vi "MergeAttrMap.vi"(6 "If exist? Skip(T)/Overwrite(F)":bool=TRUE, 8 "error in (no error)":errorcluster, 10 "AttrMap B":T1, 11 "AttrMap A":T1) -> (0 "error out":errorcluster, 3 "AttrMap A after B->A":T1)   [LabVIEW 2019, in "lv-apt-json-file.lvlib"]
uses:
  lv-apt-json-file.lvlib
  Typedef/Def-AttrMap.ctl
  f16f814e-f0a0-47f4-ae2a-f78fd01390a2.vi
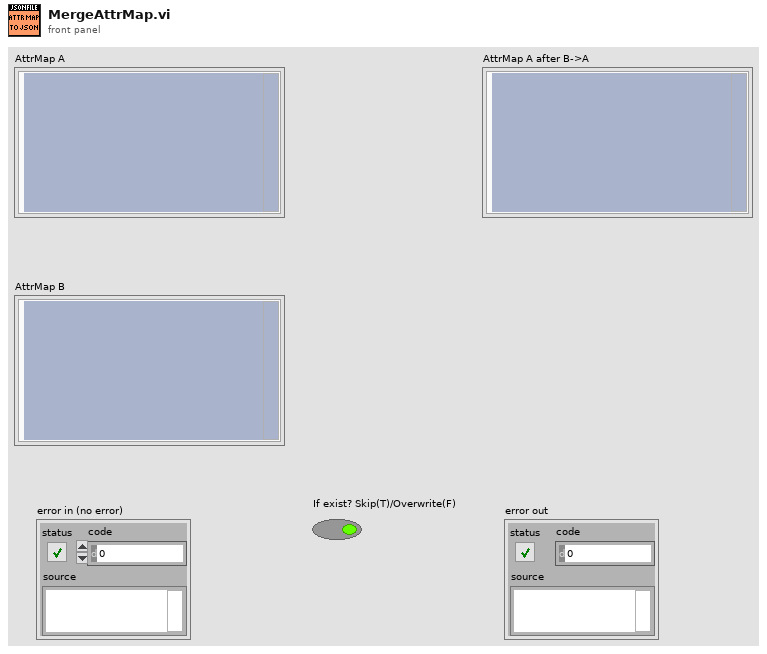
[diagram p1: front panel]
types:
  T1 = typedef "lv-apt-json-file.lvlib/Def-AttrMap.ctl" = cluster{"Map":variant}
  T2 = typedef "lv-apt-json-file.lvlib/Def-AttrMap -- Map.ctl" = map{string, string}
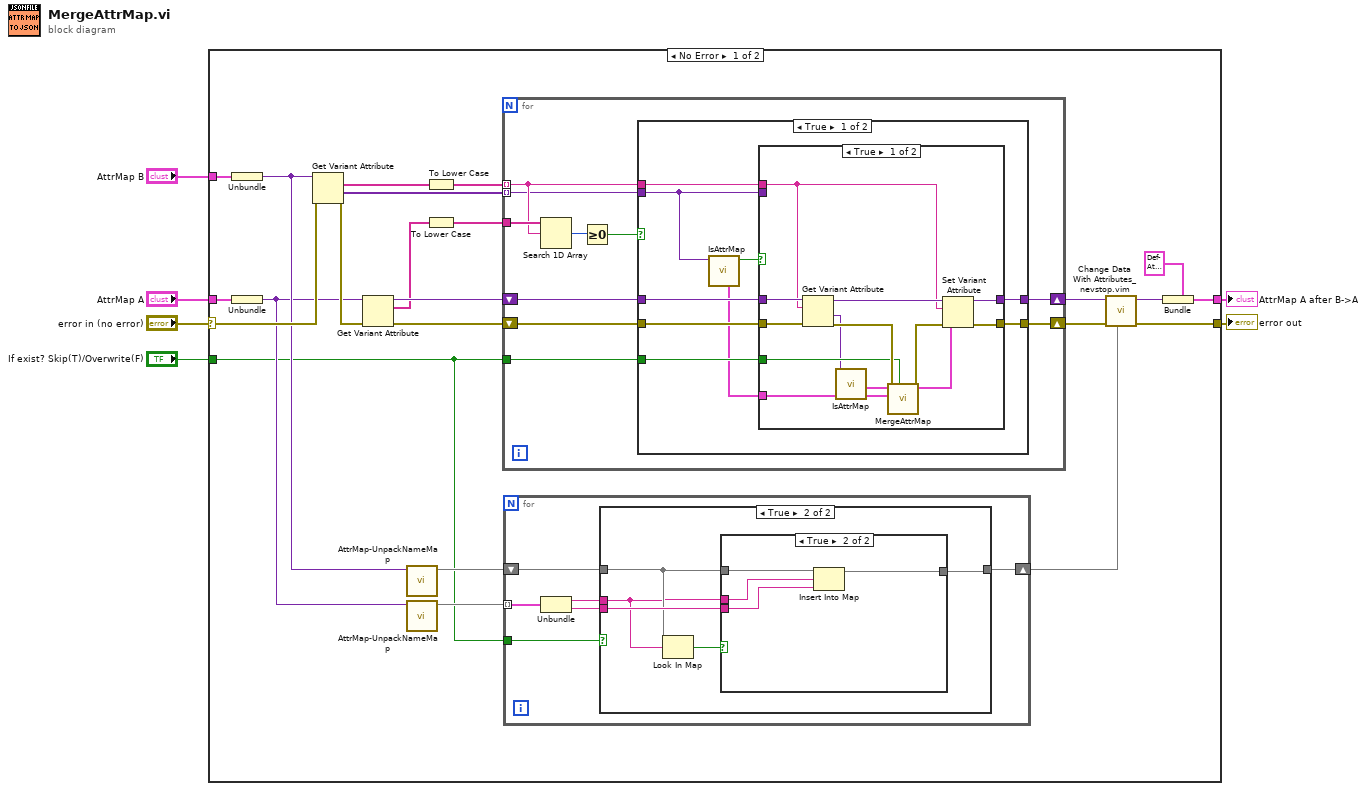
[diagram p0: block diagram]
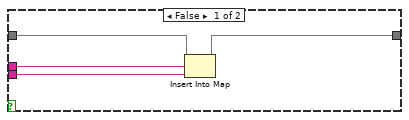
[diagram p2: hidden frame]
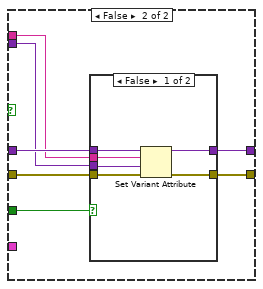
[diagram p4: hidden frame]
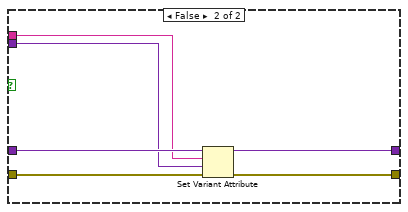
[diagram p6: hidden frame]
diagram:
  n1 = case shown="No Error" "error in (no error)" {
    selector: "error in (no error)" -> [w24 w104]
    tunnel: "AttrMap A" -> [w29 w103]
    tunnel: "AttrMap B" -> [w19 _]
    tunnel: "If exist? Skip(T)/Overwrite(F)" -> [w14 _]
    tunnel: [w9 w104] -> w2
    tunnel: [w8 w103] -> w1
    frame No Error {
      n2 = Unbundle(w19) -> ("Map"=w18:variant)
      n3 = Unbundle(w29) -> ("Map"=w17:variant)
      n4 = Get Variant Attribute(Variant=w18, error in=w24) -> (names=w21:string[], values=w22:variant[], error out=w23:errorcluster)  [unwired: 2 in, 1 out]
      n5 = Get Variant Attribute(Variant=w17, error in=w23) -> (duplicate Variant=w27:variant, names=w26:string[], error out=w28:errorcluster)  [unwired: 2 in, 1 out]
      n6 = call "AttrMap-UnpackNameMap.vi"("Map"=w18) -> ("NameMap"=w16:T2)  [unwired: 10 in]
      n7 = call "AttrMap-UnpackNameMap.vi"("Map"=w17) -> ("NameMap"=w15:T2)  [unwired: 10 in]
      n8 = To Lower Case(string=w21) -> (all lower case string=w20:string[])
      n9 = To Lower Case(string=w26) -> (all lower case string=w25:string[])
      n10 = for {
        shift-right: [w58] -> w12
        shift-left: w27 -> [w59]
        shift-right: [w56] -> w10
        shift-left: w28 -> [w57]
        tunnel: w25 -> [w55]
        tunnel: w22 -> [w51] mode=indexing
        tunnel: w20 -> [w52] mode=indexing
        tunnel: w14 -> [w50]
        n11 = Search 1D Array(1D array=w55, element=w52) -> (index of element=w54:i32)  [unwired: 1 in]
        n12 = Greater Or Equal To 0?(x=w54) -> (x >= 0?=w53:bool)
        n13 = case shown="True" w53 {
          tunnel: w59 -> [w68 w102]
          tunnel: [w67 w101] -> w58
          tunnel: w57 -> [w66 w100]
          tunnel: [w65 w99] -> w56
          tunnel: w52 -> [w62 w98]
          tunnel: w51 -> [w61 w97]
          tunnel: w50 -> [w63 _]
          frame True {
            n14 = call "IsAttrMap.vi"("Variant"=w61) -> ("True"=w64:bool, "AttrMap"=w60:T1)  [unwired: 8 in, 1 out]
            n15 = case shown="True" w64 {
              tunnel: w68 -> [w81 w88]
              tunnel: [w79 w87] -> w67
              tunnel: w66 -> [w80 w86]
              tunnel: [w78 w85] -> w65
              tunnel: w63 -> [w72 w84]
              tunnel: w62 -> [w75 w83]
              tunnel: w61 -> [_ w82]
              tunnel: w60 -> [w69 _]
              frame True {
                n16 = Get Variant Attribute(Variant=w81, name=w75, error in=w80) -> (duplicate Variant=w77:variant, value=w71:variant, error out=w74:errorcluster)  [unwired: 1 in, 1 out]
                n17 = call "IsAttrMap.vi"("Variant"=w71) -> ("AttrMap"=w70:T1)  [unwired: 8 in, 2 out]
                n18 = call "MergeAttrMap.vi"("If exist? Skip(T)/Overwrite(F)"=w72, "error in (no error)"=w74, "AttrMap B"=w69, "AttrMap A"=w70) -> ("error out"=w73:errorcluster, "AttrMap A after B->A"=w76:T1)  [unwired: 6 in]
                n19 = Set Variant Attribute(Variant=w77, name=w75, value=w76, error in=w73) -> (Variant out=w79:variant, error out=w78:errorcluster)  [unwired: 1 out]
              }
              frame False {
                n20 = case shown="False" w84 {
                  tunnel: w88 -> [w94 w96]
                  tunnel: [w93 w96] -> w87
                  tunnel: w86 -> [w92 w95]
                  tunnel: [w91 w95] -> w85
                  tunnel: w83 -> [w90 _]
                  tunnel: w82 -> [w89 _]
                  frame False {
                    n21 = Set Variant Attribute(Variant=w94, name=w90, value=w89, error in=w92) -> (Variant out=w93:variant, error out=w91:errorcluster)  [unwired: 1 out]
                  }
                  frame True {
                  }
                }
              }
            }
          }
          frame False {
            n22 = Set Variant Attribute(Variant=w102, name=w98, value=w97, error in=w100) -> (Variant out=w101:variant, error out=w99:errorcluster)  [unwired: 1 out]
          }
        }
      }
      n23 = for {
        tunnel: w15 -> [w33] mode=indexing
        shift-right: [w30] -> w13
        shift-left: w16 -> [w34]
        tunnel: w14 -> [w35]
        n24 = Unbundle(w33) -> (w32:string, w31:string)
        n25 = case shown="True" w35 {
          tunnel: w34 -> [w39 w42]
          tunnel: w32 -> [w38 w40]
          tunnel: w31 -> [w37 w43]
          tunnel: [w36 w41] -> w30
          frame False {
            n26 = Insert Into Map(map in=w39, key=w38, value=w37) -> (map out=w36:T2)  [unwired: 2 out]
          }
          frame True {
            n27 = Look In Map(map=w42, key=w40) -> (key not found?=w44:bool)  [unwired: 1 in, 1 out]
            n28 = case shown="True" w44 {
              tunnel: w43 -> [_ w47]
              tunnel: w42 -> [w45 w49]
              tunnel: [w45 w48] -> w41
              tunnel: w40 -> [_ w46]
              frame False {
              }
              frame True {
                n29 = Insert Into Map(map in=w49, key=w46, value=w47) -> (map out=w48:T2)  [unwired: 2 out]
              }
            }
          }
        }
      }
      n30 = call "Change Data With Attributes_nevstop.vim"("Data"=w13, "error in (no error)"=w10, "Variant in"=w12) -> ("error out"=w9:errorcluster, "Variant out"=w11:variant)  [unwired: 7 in]
      n31 = Bundle(cluster=T1 {"Map"=variant} ("AttrMap"), "Map"=w11) -> (w8:T1)
    }
    frame Error {
    }
  }
  "AttrMap A after B->A" <- w1
  "error out" <- w2
